vi "FG_ADS1299EVMEstyxFiles.vi"(6 "Initialization File Path":path, 8 "Read/Write (F)":bool, 9 "Storage Info":variant) -> (0 "All Files":string[](array[string]), 1 "File Path":string)   [LabVIEW 2010]
doc: "This VI serves to store and access the information regarding the estyx file structure. \n\nInputs:\nInitalization File Path - location of file read to initialize this VI.\nRead/Write (F): default FALSE\n - Read File Path for input tag (FALSE)\n - Write File info for storage (TRUE)\n\nStorage Info - variant with data in the format\n - READ mode: data is tag string for file to retrieve path for\n - WRITE mode: data is an array of clusters (cluster = file path (string) and file tag (string))\n\nOutputs:\nFile Path - \n - READ mode: estyx file path of file reference to the input\n - WRITE mode: N/A\nAll Files - array of all estyx files in storage (string array)"
uses:
  TYP_ADS1299Estyx File Enum.ctl
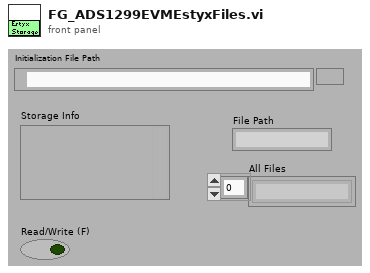
[diagram p1: front panel]
types:
  T1 = typedef "TYP_ADS1299Estyx File Enum.ctl" = enum16{"|version", "|id", "ads1299evm|blocksize_samples", "ads1299evm|acquire", "ads1299evm|data", "conf|ch1set", "conf|ch2set", "conf|ch3set", "conf|ch4set", "conf|ch5set", "conf|ch6set", "conf|ch7set", "conf|ch8set", "conf|config1", "conf|config2", "conf|config3", "conf|devid", "conf|gpio", "conf|loff", "conf|loffflip", "conf|loffsensn", "conf|loffsensp", "conf|loffstatn", "conf|loffstatp", "conf|misc2", "conf|misc1", "conf|biassensn", "conf|biassensp", "conf|reset", "conf|sleep", "conf|config4", "led|dp", "led|seg", "led|ch", "mmb0|pll", "mmb0|clkout", "mmb0|clkfreq"}
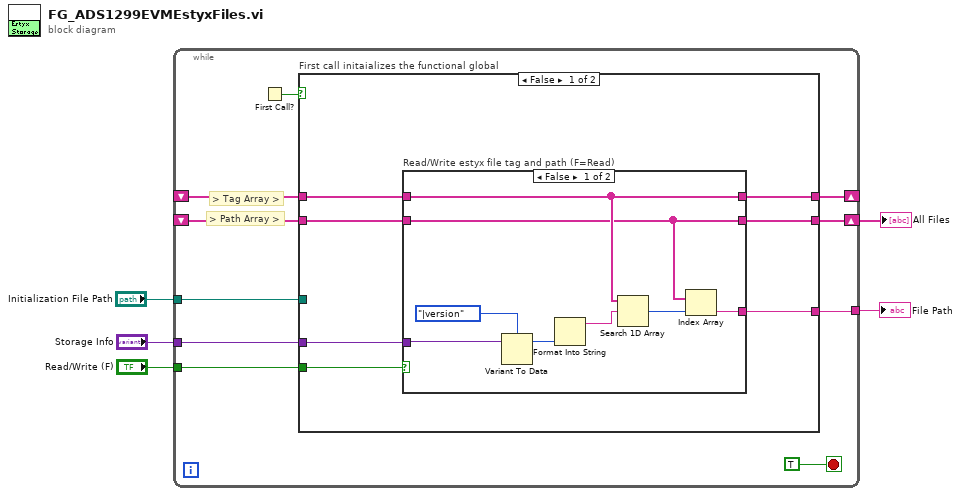
[diagram p0: block diagram]
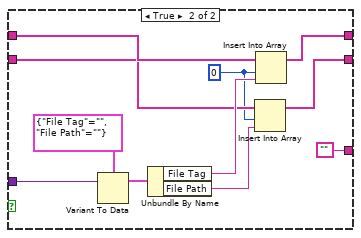
[diagram p2: hidden frame]
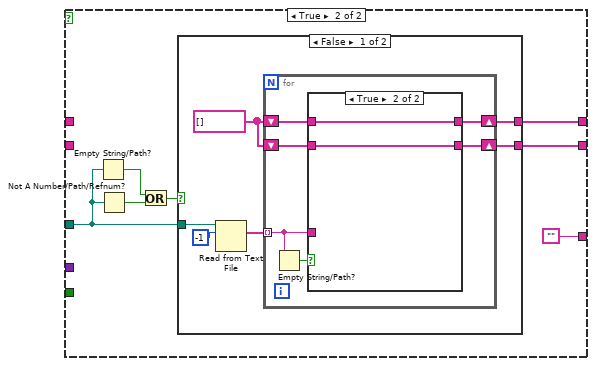
[diagram p3: hidden frame]
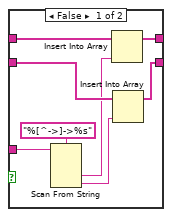
[diagram p4: hidden frame]
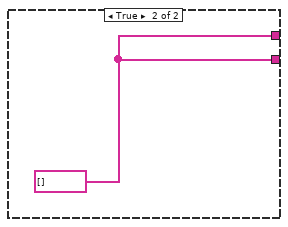
[diagram p5: hidden frame]
diagram:
  n1 = while {
    tunnel: "Read/Write (F)" -> [w14]
    shift-right: [w13] -> _
    shift-left: _ -> [w12]
    tunnel: "Storage Info" -> [w8]
    shift-right: [w10] -> w2
    shift-left: _ -> [w11]
    tunnel: [w9] -> w4
    tunnel: "Initialization File Path" -> [w6]
    stop <- TRUE stop-if-true
    # "> Path Array >"
    # "> Tag Array >"
    n2 = First Call?() -> (First Call?: T/F=w7:bool)
    n3 = case "First call initaializes the functional global" shown="False" w7 {
      tunnel: w14 -> [w22 _]
      tunnel: [w21 w47] -> w13
      tunnel: w12 -> [w20 _]
      tunnel: w11 -> [w19 _]
      tunnel: [w18 w46] -> w10
      tunnel: [w17 ""] -> w9
      tunnel: w8 -> [w16 _]
      tunnel: w6 -> [_ w45]
      frame False {
        n4 = case "Read/Write estyx file tag and path (F=Read)" shown="False" w22 {
          tunnel: [w30 w41] -> w21
          tunnel: w20 -> [w30 w40]
          tunnel: w19 -> [w29 w37]
          tunnel: [w29 w36] -> w18
          tunnel: [w27 ""] -> w17
          tunnel: w16 -> [w26 w32]
          frame False {
            n5 = Variant To Data(Variant=w26, type=TYP_ADS1299Estyx_File_Enum."|version" ("Styx File Tags - Enum")) -> (data=w25:T1)  [unwired: 1 in, 1 out]
            n6 = Format Into String(w25) -> (resulting string=w24:string)  [unwired: 3 in, 1 out]
            n7 = Search 1D Array(1D array=w30, element=w24) -> (index of element=w28:i32)  [unwired: 1 out]
            n8 = Index Array(array=w29, index=w28) -> (element=w27:string)
          }
          frame True {
            w35 = 0
            n9 = Variant To Data(Variant=w32, type=cluster{"File Tag":string, "File Path":string} {"File Tag"="", "File Path"=""} ("Estyx File Info")) -> (data=w33:cluster{"File Tag":string, "File Path":string})  [unwired: 1 in, 1 out]
            n10 = Unbundle By Name(w33) -> ("File Tag"=w39:string, "File Path"=w38:string)
            n11 = Insert Into Array(array=w37, index=w35, new element=w38) -> (w36:string[])
            n12 = Insert Into Array(array=w40, index=w35, new element=w39) -> (w41:string[])
          }
        }
      }
      frame True {
        n13 = Empty String/Path?(string/path=w45) -> (empty?=w42:bool)
        n14 = Not A Number/Path/Refnum?(number/path/refnum=w45) -> (NaN/Path/Refnum?=w43:bool)
        n15 = Or(x=w42, y=w43) -> (x .or. y?=w44:bool)
        n16 = case shown="False" w44 {
          tunnel: [w52 w71] -> w47
          tunnel: [w51 w71] -> w46
          tunnel: w45 -> [w50 _]
          frame False {
            w49 = string[] []
            n17 = Read from Text File(file (use dialog)=w50, count=-1) -> (text=w53:string[])  [unwired: 1 in, 4 out]
            n18 = for {
              tunnel: w53 -> [w55] mode=indexing
              shift-right: [w58] -> w52
              shift-left: w49 -> [w60]
              shift-right: [w57] -> w51
              shift-left: w49 -> [w59]
              n19 = Empty String/Path?(string/path=w55) -> (empty?=w56:bool)
              n20 = case shown="True" w56 {
                tunnel: w55 -> [w68 _]
                tunnel: w60 -> [w65 w70]
                tunnel: w59 -> [w64 w69]
                tunnel: [w66 w70] -> w58
                tunnel: [w63 w69] -> w57
                frame False {
                  n21 = Scan From String(format string="%[^->]->%s", input string=w68) -> (output 1=w62:string, output 2=w61:string)  [unwired: 2 in, 5 out]
                  n22 = Insert Into Array(array=w65, new element=w62) -> (w66:string[])  [unwired: 1 in]
                  n23 = Insert Into Array(array=w64, new element=w61) -> (w63:string[])  [unwired: 1 in]
                }
                frame True {
                }
              }
            }
          }
          frame True {
            w71 = string[] []
          }
        }
      }
    }
  }
  "File Path" <- w4
  "All Files" <- w2
